vi "Cascade setup camera new.vi"(0 "ADC speed":i32=-2 min=-3 step=1, 1 "Exposure":dbl, 3 "Clocking parameters":T1={"Clear mode"=2, "# clear cycles"=2, "Clocking mode"=1} {"Clocking mode" items=["Normal", "Frame-transfer"]; "Clear mode" items=["Don't clear", "Clear pre-exposure", "Clear pre-sequence", "Clear post-sequence", "Clear pre- and post-sequence", "Clear pre-exposure and post-sequence"]}, 5 "ADC Gain":i32=-1 min=-1 step=1, 7 "ADC Offset":i32=-1 min=-1 step=1, 9 "Readout Port":i32=-1 min=-1 step=1, 11 "error in (no error)":errorcluster, 12 "EM Gain":u16, 13 "ROI":T2={"X Start"=1, "X End"=1, "X Bin"=1, "Y Start"=1, "Y End"=1, "Y Bin"=1} {"Y Bin" min=1 step=1; "Y End" min=1 step=1; "Y Start" min=1 step=1; "X Bin" min=1 step=1; "X End" min=1 step=1; "X Start" min=1 step=1}) -> (6 "ADC Parameters":T3, 8 "Exposure time":dbl format="%.2f", 10 "EM Parameters":cluster{"Enabled?":dbl, "Gain":dbl}, 15 "error out (no error)":errorcluster)   [LabVIEW 2011]
doc: "Copyright (c) 2004-2006 Jeff Gelles Brandeis University"
uses:
  Cascade-specific globals.vi
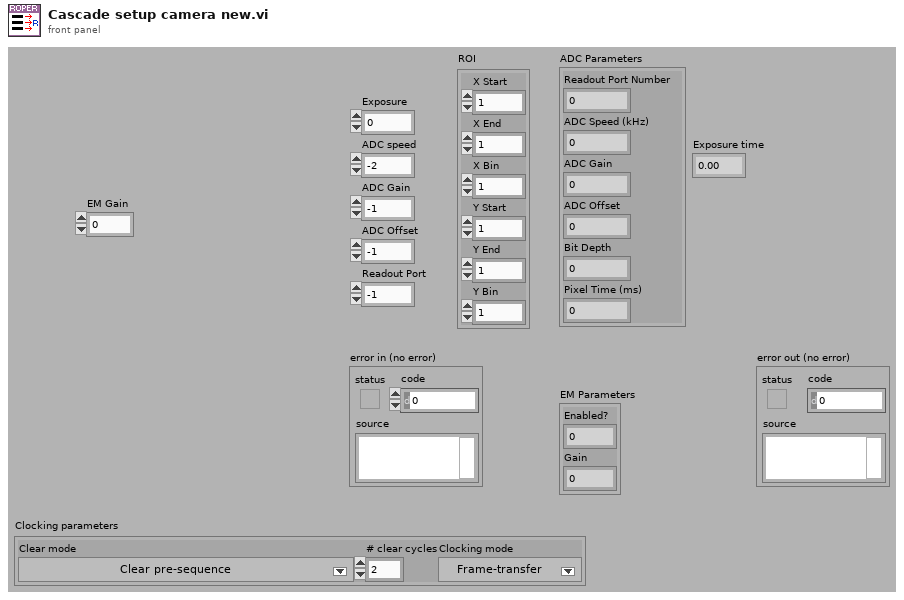
[diagram p1: front panel]
types:
  T1 = cluster{"Clear mode":u8, "# clear cycles":u16, "Clocking mode":u8}
  T2 = cluster{"X Start":u32, "X End":u32, "X Bin":u32, "Y Start":u32, "Y End":u32, "Y Bin":u32}
  T3 = cluster{"Readout Port Number":i32, "ADC Speed (kHz)":i32, "ADC Gain":i32, "ADC Offset":i32, "Bit Depth":i32, "Pixel Time (ms)":i32}
  T4 = cluster{"Camera Handle":u32, "Pulser Handle":u32, "File Handle":u32, "Display Handle":u32, "Image Handle":u32}
  T5 = cluster{"acquire Mode":u32, "Exposure":dbl, "Number of frames\n0 = continuous":u32, "Software Accumulations":u32}
  T6 = cluster{"Readout Port":i32, "ADC Speed":i32, "ADC Gain":i32, "ADC Offset":i32, "Bit Depth":i32, "Pixel Time":i32}
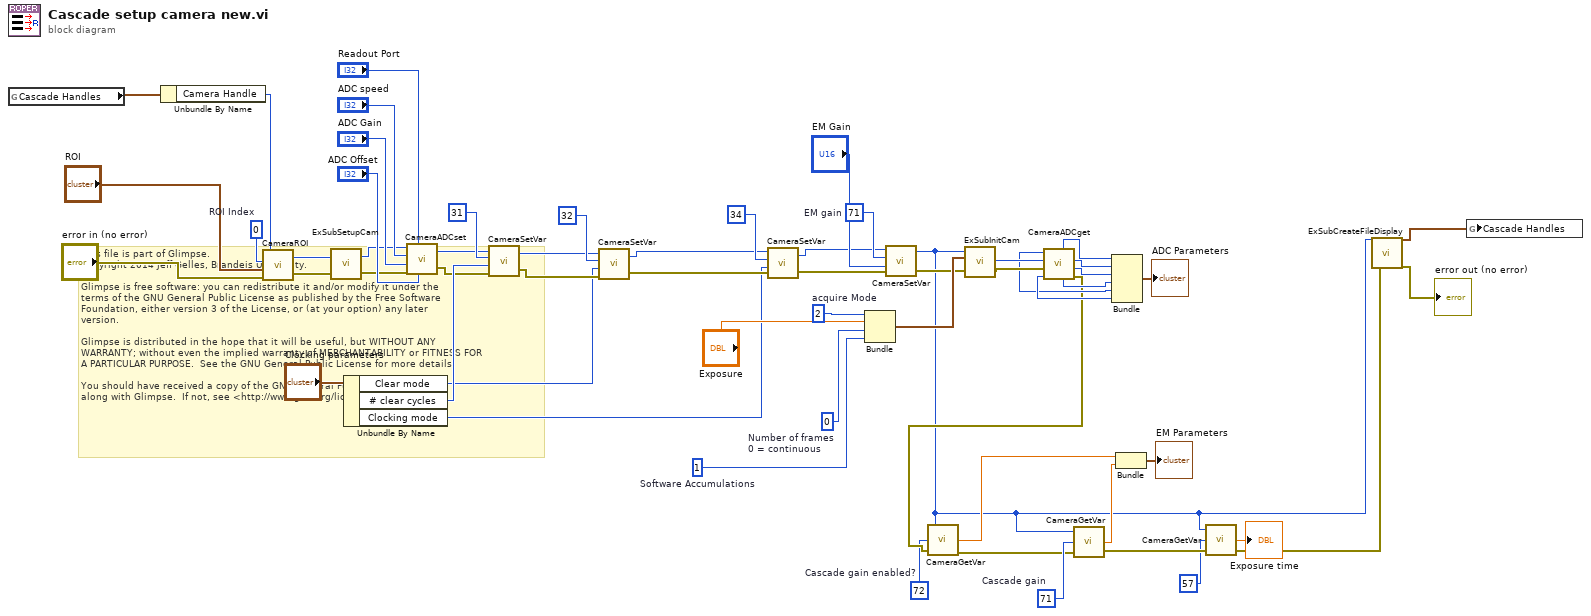
[diagram p0: block diagram]
diagram:
  w8 = u32 0  # ROI Index
  w36 = u32 71  # EM gain
  w42 = u32 71  # Cascade gain
  w43 = u32 72  # Cascade gain enabled?
  w54 = u32 2  # acquire Mode
  w55 = u32 0  # Number of frames 0 = continuous
  w56 = u32 1  # Software Accumulations
  # "This file is part of Glimpse. \nCopyright 2014 Jeff Gelles, Brandeis University.    \n\nGlimpse is free software: you can redistribute it and/or modify it under the \nterms of the GNU General Public License as published by the Free Software \nFoundation, either version 3 of the License, or (at your option) any later \nversion.\n\nGlimpse is distributed in the hope that it will be useful, but WITHOUT ANY \nWARRANTY; without even the implied warranty of MERCHANTABILITY or FITNESS FOR \nA PARTICULAR PURPOSE.  See the GNU General Public License for more details.\n\nYou should have received a copy of the GNU General Public License\nalong with Glimpse.  If not, see <http://www.gnu.org/licenses/>."
  n1 = global read "Cascade-specific globals.vi" "Cascade Handles"() -> (w5:T4)
  n2 = Unbundle By Name(w5) -> ("Camera Handle"=w4:u32)
  n3 = call <userlib>:"CameraROI.vi"("error in"="error in (no error)", "ROI Params"="ROI", "ROI Index"=w8, "Camera Handle"=w4) -> ("error out"=w3:errorcluster, "Camera Handle"=w2:u32)
  n4 = call "ExSubSetupCam.vi"("error in (no error)"=w3, "Camera Handle"=w2) -> ("error out"=w30:errorcluster, "Camera Handle"=w29:u32)
  n5 = Unbundle By Name("Clocking parameters") -> ("Clear mode"=w15:u8, "# clear cycles"=w20:u16, "Clocking mode"=w14:u8)
  n6 = call <userlib>:"CameraADCset.vi"("ADC offset"="ADC Offset", "Read Out port"="Readout Port", "error in (no error)"=w30, "ADC Gain"="ADC Gain", "ADC Speed"="ADC speed", "Camera Handle"=w29) -> ("error out"=w19:errorcluster, "Camera Handle"=w25:u32)
  n7 = call <userlib>:"CameraSetVar.vi"("error in"=w19, "Value"=w20, "Parameter ID"=u32 31 ("# clear cycles"), "Camera Handle"=w25) -> ("error out"=w18:errorcluster, "CameraHandle"=w24:u32)
  n8 = call <userlib>:"CameraSetVar.vi"("error in"=w18, "Value"=w15, "Parameter ID"=u32 32 ("EM gain"), "Camera Handle"=w24) -> ("error out"=w17:errorcluster, "CameraHandle"=w23:u32)
  n9 = call <userlib>:"CameraSetVar.vi"("error in"=w17, "Value"=w14, "Parameter ID"=u32 34 ("EM gain"), "Camera Handle"=w23) -> ("error out"=w16:errorcluster, "CameraHandle"=w22:u32)
  n10 = Bundle("acquire Mode"=w54, "Exposure"="Exposure", "Number of frames\n0 = continuous"=w55, "Software Accumulations"=w56) -> (w58:T5)  [unwired: 1 out]
  n11 = call <userlib>:"CameraSetVar.vi"("error in"=w16, "Value"="EM Gain", "Parameter ID"=w36, "Camera Handle"=w22) -> ("error out"=w37:errorcluster, "CameraHandle"=w11:u32)
  n12 = call "ExSubInitCam.vi"("error in (no error)"=w37, "Camera Information"=w58, "Camera Handle"=w11) -> ("error out"=w52:errorcluster, "Camera Handle"=w53:u32)
  n13 = call <userlib>:"CameraADCget.vi"("Camera handle"=w53, "error in (no error)"=w52) -> ("Bit Depth"=w46:i32, "Pixel Time"=w47:i32, "Readout Port"=w51:i32, "ADC Offset"=w48:i32, "ADC Speed"=w50:i32, "ADC Gain"=w49:i32, "error out"=w44:errorcluster)  [unwired: 1 out]
  n14 = call <userlib>:"CameraGetVar.vi"("error in"=w44, "Parameter ID"=w43, "Camera Handle"=w11) -> ("error out"=w41:errorcluster, "Value"=w40:dbl)  [unwired: 1 out]
  n15 = call <userlib>:"CameraGetVar.vi"("error in"=w41, "Parameter ID"=w42, "Camera Handle"=w11) -> ("error out"=w13:errorcluster, "Value"=w39:dbl)  [unwired: 1 out]
  n16 = Bundle("Readout Port"=w51, "ADC Speed"=w50, "ADC Gain"=w49, "ADC Offset"=w48, "Bit Depth"=w46, "Pixel Time"=w47) -> (→"ADC Parameters":T6)  [unwired: 1 out]
  n17 = Bundle("Value"=w40, "Value"=w39) -> (→"EM Parameters":cluster{"Value":dbl, "Value":dbl})  [unwired: 1 out]
  n18 = call <userlib>:"CameraGetVar.vi"("error in"=w13, "Parameter ID"=u32 57, "Camera Handle"=w11) -> ("error out"=w12:errorcluster, "Value"=→"Exposure time":dbl)  [unwired: 1 out]
  n19 = call "ExSubCreateFileDisplay.vi"("error in (no error)"=w12, "Camera Handle"=w11) -> ("error out"=→"error out (no error)":errorcluster, "Handles Out"=w1:T4)  [unwired: 2 in]
  n20 = global write "Cascade-specific globals.vi" "Cascade Handles"(w1) -> ()
